vi "Sensible Tab Order.vi"(11 "Bool Refnum":refnum<vi>) -> ()   [LabVIEW 2012]
doc: "When placed in the block diagram of a VI, this subVI makes tabbing ignore clusters, rather than getting stuck inside of them. Tabbing will automatically enter a cluster, follow the cluster's order, and then exit it and proceed as normal. A refnum to a boolean must be provided so that this subVI knows when to exit; it will exit on a value change event.\n\n<B>Note: this must be used as a subVI.</B>"
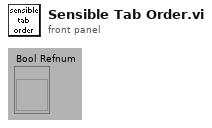
[diagram p1: front panel]
types:
  T1 = cluster{"Shift":bool, "Ctrl":bool, "Alt":bool, "Cmd":bool, "Opt":bool}
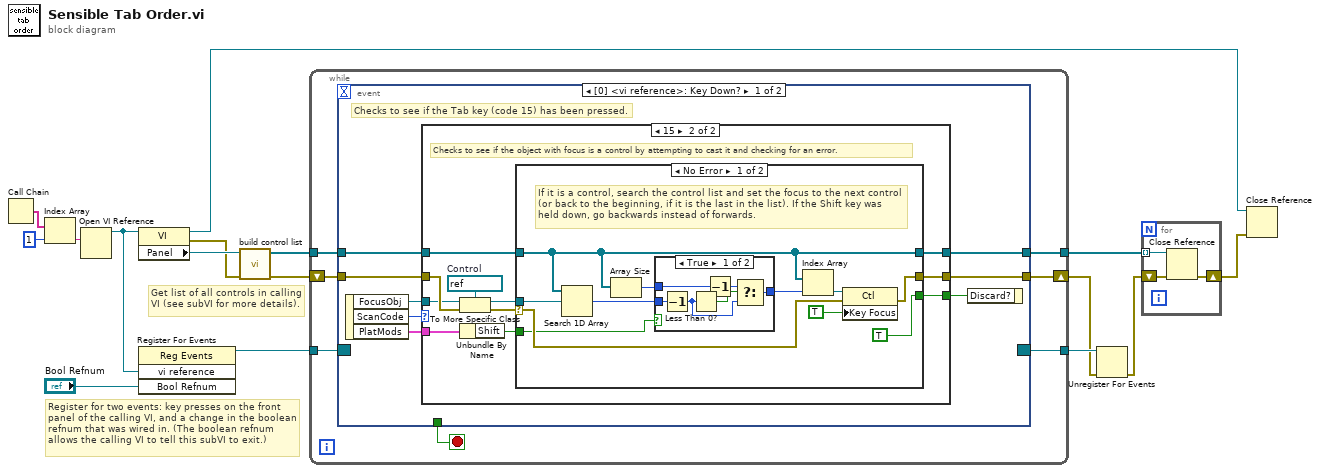
[diagram p0: block diagram]
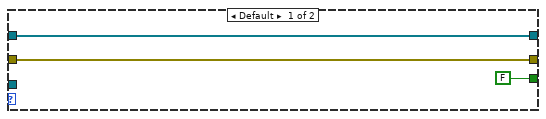
[diagram p2: hidden frame]
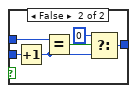
[diagram p3: hidden frame]
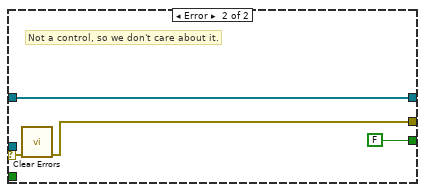
[diagram p4: hidden frame]
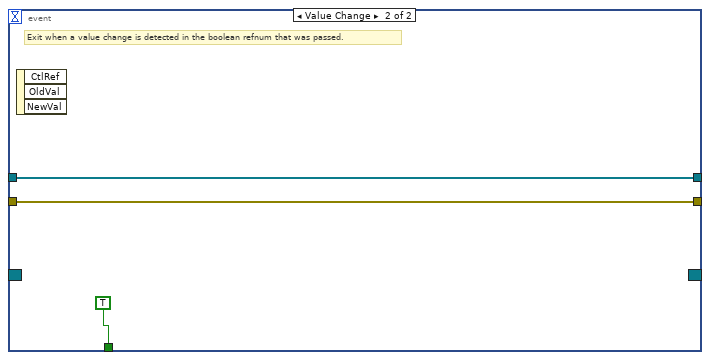
[diagram p5: hidden frame]
diagram:
  # "Get list of all controls in calling VI (see subVI for more details)."
  # "Register for two events: key presses on the front panel of the calling VI, and a change in the boolean refnum that was wired in. (The boolean refnum allows the calling VI to tell this subVI to exit.)"
  n1 = Call Chain() -> (call chain=w12:string[])
  n2 = Index Array(array=w12, index=1) -> (element=w10:string)
  n3 = Open VI Reference(vi path=w10) -> (vi reference=w9:refnum<vi>)  [unwired: 1 in, 5 out]
  n4 = property class="VI"(reference=w9) -> (reference out=w13:refnum<vi>, error out=w5:errorcluster, "Panel"=w6:refnum<vi>)  [unwired: 1 in]
  n5 = register-events(w9, "Bool Refnum") -> (reference out=w8:refnum<event-registration>)  [unwired: 2 in, 1 out]
  n6 = call "build control list.vi"("error in (no error)"=w5, "Generic Refnum"=w6) -> ("error out"=w15:errorcluster, "Controls[] list"=w16:refnum<vi>[])  [unwired: 8 out]
  n7 = while {
    tunnel: w16 -> [w22]
    shift-right: [w20] -> w2
    shift-left: w15 -> [w21]
    tunnel: [w19] -> w14
    tunnel: w8 -> [w18]
    tunnel: [w17] -> w3
    stop <- w23 stop-if-true
    n8 = event shown="[0] <vi reference>: Key Down?" {
      selector: w18 -> [_ _]
      dyn-events: [_ _] -> w17
      timeout: _ -> [_ _]
      tunnel: [_ TRUE ("stop")] -> w23
      tunnel: w22 -> [w30 w75]
      tunnel: w21 -> [w29 w74]
      tunnel: [w27 w75] -> w19
      tunnel: [w26 w74] -> w20
      event Key Down? {
        # "Checks to see if the Tab key (code 15) has been pressed."
        n9 = event-data() -> ("FocusObj"=w28:refnum<vi>, "ScanCode"=w31:i16, "PlatMods"=w25:T1)  [unwired: 1 out]
        n10 = case shown="15" w31 {
          tunnel: w30 -> [w34 w42]
          tunnel: w29 -> [w33 w41]
          tunnel: w28 -> [_ w40]
          tunnel: [w34 w39] -> w27
          tunnel: [w33 w38] -> w26
          tunnel: w25 -> [_ w37]
          tunnel: [FALSE w35] -> w24
          frame Default {
          }
          frame 15 {
            w45 = refnum<vi> refnum  # Control
            # "Checks to see if the object with focus is a control by attempting to cast it and checking for an error."
            n11 = To More Specific Class(target class=w45, reference=w40, error in=w41) -> (specific class reference=w43:refnum<vi>, error out=w44:errorcluster)
            n12 = Unbundle By Name(w37) -> ("Shift"=w36:bool)
            n13 = case shown="No Error" w44 {
              selector: w44 -> [w50 w72]
              tunnel: w43 -> [w56 _]
              tunnel: w42 -> [w49 w71]
              tunnel: [w49 w71] -> w39
              tunnel: [w48 w70] -> w38
              tunnel: w36 -> [w47 _]
              tunnel: [TRUE FALSE] -> w35
              frame No Error {
                # "If it is a control, search the control list and set the focus to the next control (or back to the beginning, if it is the last in the list). If the Shift key was held down, go backwards instead of forwards."
                n14 = Search 1D Array(1D array=w49, element=w56) -> (index of element=w55:i32)  [unwired: 1 out]
                n15 = Array Size(array=w49) -> (size(s)=w52:i32)
                n16 = case shown="True" w47 {
                  tunnel: w55 -> [w62 w68]
                  tunnel: w52 -> [w59 w67]
                  tunnel: [w61 w64] -> w51
                  frame True {
                    n17 = Decrement(x=w62) -> (x-1=w57:i32)
                    n18 = Less Than 0?(x=w57) -> (x < 0?=w60:bool)
                    n19 = Decrement(x=w59) -> (x-1=w58:i32)
                    n20 = Select(t=w58, s=w60, f=w57) -> (s? t:f=w61:i32)
                  }
                  frame False {
                    n21 = Increment(x=w68) -> (x+1=w65:i32)
                    n22 = Equal?(x=w67, y=w65) -> (x = y?=w66:bool)
                    n23 = Select(t=0, s=w66, f=w65) -> (s? t:f=w64:i32)
                  }
                }
                n24 = Index Array(array=w49, index=w51) -> (element=w54:refnum<vi>)
                n25 = property class="Ctl"(reference=w54, error in=w50, "Key Focus"=TRUE) -> (error out=w48:errorcluster)  [unwired: 1 out]
              }
              frame Error {
                # "Not a control, so we don't care about it."
                n26 = call <vilib>:"Clear Errors.vi"("error in (no error)"=w72) -> ("error out"=w70:errorcluster)  [unwired: 6 out]
              }
            }
          }
        }
        n27 = event-data("Discard?"=w24) -> ()  [unwired: 1 in, 1 out]
      }
      event Value Change {
        # "Exit when a value change is detected in the boolean refnum that was passed."
        n28 = event-data() -> ()  [unwired: 4 out]
      }
    }
  }
  n29 = Unregister For Events(event registration refnum=w3, error in=w2) -> (error out=w1:errorcluster)
  n30 = for {
    tunnel: w14 -> [w78] mode=indexing
    shift-right: [w76] -> w4
    shift-left: w1 -> [w77]
    n31 = Close Reference(reference=w78, error in (no error)=w77) -> (error out=w76:errorcluster)
  }
  n32 = Close Reference(reference=w13, error in (no error)=w4) -> ()  [unwired: 1 out]
